vi "Get Trigger Style.vi"(8 "error in (no error)":errorcluster) -> (0 "error out":errorcluster, 3 "function return":u32)   [LabVIEW 2021, in "vmmsolib.lvlib"]
doc: "DLL_API unsigned int WINAPI GetTriggerStyle();"
uses:
  vmmsolib.lvlib
  vmmso.dll
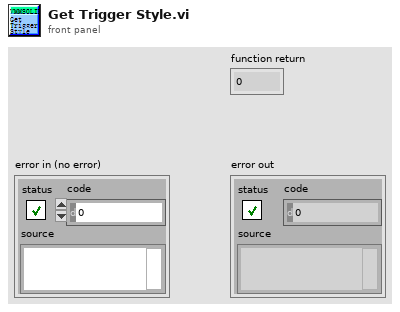
[diagram p1: front panel]
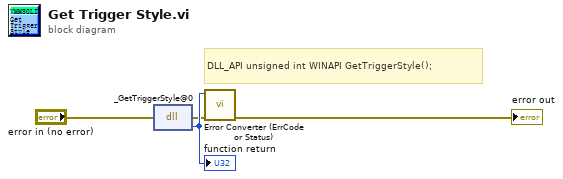
[diagram p0: block diagram]
diagram:
  # "DLL_API unsigned int WINAPI GetTriggerStyle();"
  n1 = dll-call lib="D:/VmMsoSDK/demo-Labview/2021/vmmsolib/vmmso.*" fn="_GetTriggerStyle@0"(error in="error in (no error)") -> (error out=w2:errorcluster, w4:u32)  [unwired: 2 in, 1 out]
  "function return" <- w4
  n2 = call "Error Converter (ErrCode or Status).vi"("error in (no error)"=w2, "error code"=w4) -> ("error out"=→"error out":errorcluster)  [unwired: 9 in]
